vi "Default_odour_bottles.vi"() -> (0 "Array":T1(array[cluster]))   [LabVIEW 2016]
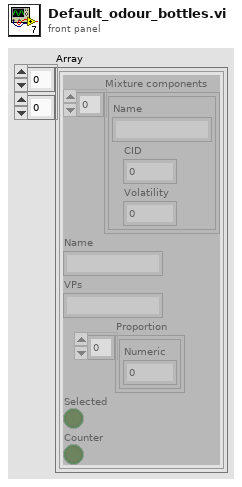
[diagram p1: front panel]
types:
  T1 = cluster{"Mixture components":cluster{"Name":string, "CID":i32, "Volatility":dbl}[], "Name":string, "VPs":string, "Proportion":cluster{"Numeric":dbl}[], "Selected":bool, "Counter":bool}[][]
  T2 = cluster{"Name":string, "CID":i32, "Volatility":dbl}[]
  T3 = cluster{"Mixture components":cluster{"Name":string, "CID":i32, "Volatility":dbl}[], "Name":string, "VPs":string, "Proportion":cluster{"Numeric":dbl}[], "Selected":bool, "Counter":bool}
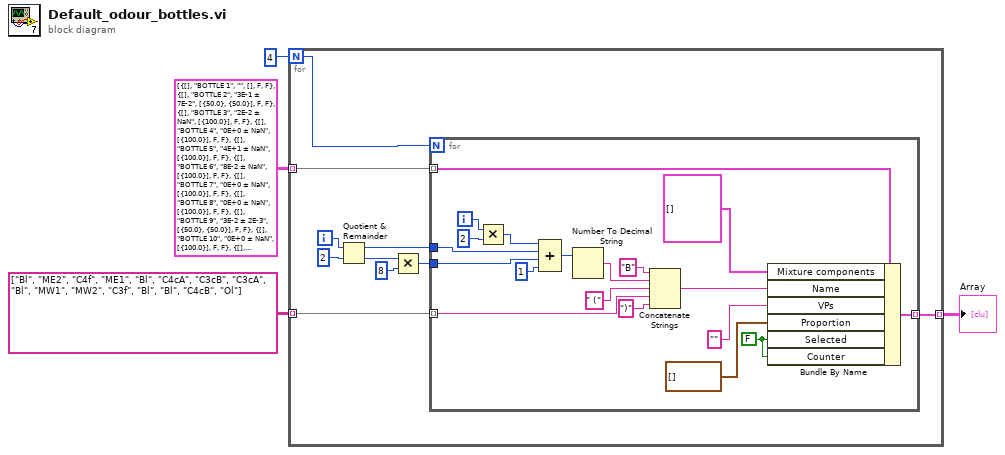
[diagram p0: block diagram]
diagram:
  n1 = for {
    N: 4 -> [w14]
    tunnel: T1 [[{"Mixture components"=[], "Name"="BOTTLE 1", "VPs"="", "Proportion"=[], "Selected"=FALSE, "Counter"=FALSE}, {"Mixture components"=[], "Name"="BOTTLE 2", "VPs"="3E-1 ± 7E-2", "Proportion"=[{"Numeric"=50.0}, {"Numeric"=50.0}], "Selected"=FALSE, "Counter"=FALSE}, {"Mixture components"=[], "Name"="BOTTLE 3", "VPs"="2E-2 ± NaN", "Proportion"=[{"Numeric"=100.0}], "Selected"=FALSE, "Counter"=FALSE}, {"Mixture components"=[], "Name"="BOTTLE 4", "VPs"="0E+0 ± NaN", "Proportion"=[{"Numeric"=100.0}], "Selected"=FALSE, "Counter"=FALSE}], [{"Mixture components"=[], "Name"="BOTTLE 5", "VPs"="4E+1 ± NaN", "Proportion"=[{"Numeric"=100.0}], "Selected"=FALSE, "Counter"=FALSE}, {"Mixture components"=[], "Name"="BOTTLE 6", "VPs"="8E-2 ± NaN", "Proportion"=[{"Numeric"=100.0}], "Selected"=FALSE, "Counter"=FALSE}, {"Mixture components"=[], "Name"="BOTTLE 7", "VPs"="0E+0 ± NaN", "Proportion"=[{"Numeric"=100.0}], "Selected"=FALSE, "Counter"=FALSE}, {"Mixture components"=[], "Name"="BOTTLE 8", "VPs"="0E+0 ± NaN", "Proportion"=[{"Numeric"=100.0}], "Selected"=FALSE, "Counter"=FALSE}], [{"Mixture components"=[], "Name"="BOTTLE 9", "VPs"="3E-2 ± 2E-3", "Proportion"=[{"Numeric"=50.0}, {"Numeric"=50.0}], "Selected"=FALSE, "Counter"=FALSE}, {"Mixture components"=[], "Name"="BOTTLE 10", "VPs"="0E+0 ± NaN", "Proportion"=[{"Numeric"=100.0}], "Selected"=FALSE, "Counter"=FALSE}, {"Mixture components"=[], "Name"="BOTTLE 11", "VPs"="5E-2 ± 3E-2", "Proportion"=[{"Numeric"=50.0}, {"Numeric"=50.0}], "Selected"=FALSE, "Counter"=FALSE}, {"Mixture components"=[], "Name"="BOTTLE 12", "VPs"="4E+0 ± NaN", "Proportion"=[{"Numeric"=100.0}], "Selected"=FALSE, "Counter"=FALSE}], [{"Mixture components"=[], "Name"="BOTTLE 13", "VPs"="3E+1 ± NaN", "Proportion"=[{"Numeric"=100.0}], "Selected"=FALSE, "Counter"=FALSE}, {"Mixture components"=[], "Name"="BOTTLE 14", "VPs"="0E+0 ± NaN", "Proportion"=[{"Numeric"=100.0}], "Selected"=FALSE, "Counter"=FALSE}, {"Mixture components"=[], "Name"="BOTTLE 15", "VPs"="2E-2 ± NaN", "Proportion"=[{"Numeric"=100.0}], "Selected"=FALSE, "Counter"=FALSE}, {"Mixture components"=[], "Name"="BOTTLE 16", "VPs"="7E-1 ± NaN", "Proportion"=[{"Numeric"=100.0}], "Selected"=FALSE, "Counter"=FALSE}]] ("Array") -> [w13] mode=indexing
    tunnel: [w12] -> w1 mode=indexing
    tunnel: string[][] [["Bl", "ME2", "C4f", "ME1"], ["Bl", "C4cA", "C3cB", "C3cA"], ["Bl", "MW1", "MW2", "C3f"], ["Bl", "Bl", "C4cB", "Ol"]] -> [w11] mode=indexing
    i -> [w10]
    n2 = Quotient & Remainder(x=w10, y=2) -> (x-y*floor(x/y)=w5:i32, floor(x/y)=w8:i32)
    n3 = Multiply(x=w8, y=8) -> (x*y=w6:i32)
    n4 = for {
      N: w14 -> [_]
      tunnel: w13 -> [w33] mode=indexing
      tunnel: [w29] -> w12 mode=indexing
      tunnel: w11 -> [w25] mode=indexing
      tunnel: w6 -> [w21]
      tunnel: w5 -> [w20]
      i -> [w19]
      w22 = FALSE ("Selected")
      n5 = Multiply(x=w19, y=2) -> (x*y=w17:i32)
      n6 = Compound Arithmetic op=ADD(w17, w20, w21, 1 ("value")) -> (w16:i32)
      n7 = Number To Decimal String(number=w16) -> (decimal integer string=w32:string)  [unwired: 1 in]
      n8 = Concatenate Strings("B" ("string"), w32, " (" ("string"), w25, ")" ("string")) -> (w30:string)
      n9 = Bundle By Name(cluster=w33, "Mixture components"=T2 [], "Name"=w30, "VPs"="", "Proportion"=cluster{"Numeric":dbl}[] [], "Selected"=w22, "Counter"=w22) -> (w29:T3)
    }
  }
  "Array" <- w1
